vi "Initialize.vi"(8 "error in":errorcluster, 11 "custom device reference in":T1 format="%.0x") -> (0 "error out":errorcluster, 3 "custom device reference out":T1 format="%.0x")   [LabVIEW 2020, in "Ballard ARINC 429 System Explorer.lvlib" / "Implementation.lvlib"]
uses:
  Implementation.lvlib
  <vilib>/NI VeriStand/Custom Device API/Custom Device Item Ref.ctl
  Shared/Device Parameters.ctl
  Shared/Initialization Method.ctl
  Scripting/Constants.vi
  <vilib>/NI VeriStand/Custom Device API/Set Item Property (Boolean).vi
  Scripting/Ballard ARINC 429 Scripting.lvlib
  <vilib>/NI VeriStand/Custom Device API/Custom Device API.lvlib
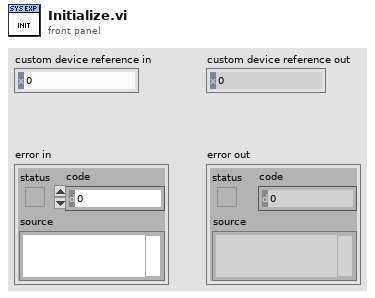
[diagram p1: front panel]
types:
  T1 = typedef "Custom Device API.lvlib/Custom Device Item Ref.ctl" = u64
  T2 = typedef "Device Parameters.ctl" = cluster{"initialization method":T3, "card number":i32, "PXI slot number":i32, "core number":i32}
  T3 = typedef "Initialization Method.ctl" = enum16{"PXI Slot Number", "Card Number"}
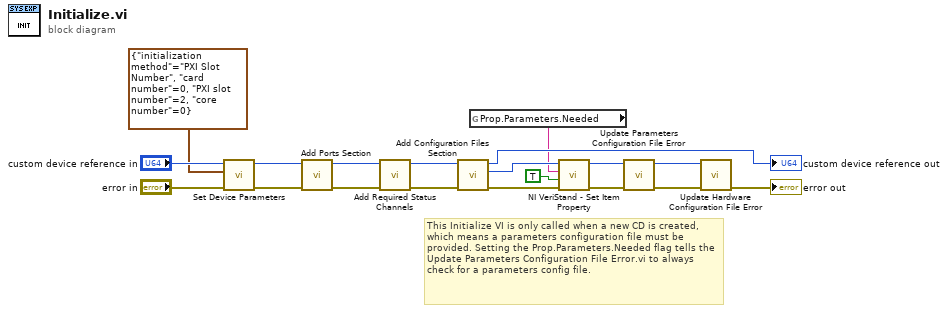
[diagram p0: block diagram]
diagram:
  # "This Initialize VI is only called when a new CD is created, which means a parameters configuration file must be provided. Setting the Prop.Parameters.Needed flag tells the Update Parameters Configuration File Error.vi to always check for a parameters config file."
  n1 = call "Set Device Parameters.vi"("error in"="error in", "device parameters"=T2 {"initialization method"=enum."PXI Slot Number", "card number"=0, "PXI slot number"=2, "core number"=0}, "Ballard ARINC 429 custom device in"="custom device reference in") -> ("error out"=w6:errorcluster, "Ballard ARINC 429 custom device out"=w7:T1)  [unwired: 7 in]
  n2 = call "Add Ports Section.vi"("error in"=w6, "custom device ref"=w7) -> ("error out"=w3:errorcluster, "custom device ref out"=w4:T1)  [unwired: 7 in, 1 out]
  n3 = call "Add Required Status Channels.vi"("error in"=w3, "custom device reference"=w4) -> ("error out"=w1:errorcluster, "custom device reference out"=w2:T1)  [unwired: 7 in, 1 out]
  n4 = call "Add Configuration Files Section.vi"("error in"=w1, "Custom device Ref"=w2) -> ("error out"=w18:errorcluster, "Configuration files Ref"=w16:T1, "Custom device Ref out"=→"custom device reference out":T1)  [unwired: 7 in]
  n5 = global read "Constants.vi" "Prop.Parameters.Needed"() -> (w13:string)
  n6 = call-poly <vilib>:"NI VeriStand - Set Item Property.vi"("error in (no error)"=w18, "Value"=TRUE, "Property Name"=w13, "Item Ref in"=w16) -> ("error out"=w17:errorcluster, "Item Ref out"=w15:T1)  [unwired: 5 in, 1 out]
  n7 = call "Update Parameters Configuration File Error.vi"("error in"=w17, "Configuration files Ref"=w15) -> ("error out"=w12:errorcluster, "Configuration files Ref out"=w10:T1)  [unwired: 8 in]
  n8 = call "Update Hardware Configuration File Error.vi"("error in"=w12, "Configuration files Ref"=w10) -> ("error out"=→"error out":errorcluster)  [unwired: 8 in, 1 out]
